vi "TEST - Main Editor VI Not Broken.vi"() -> (0 "error out":errorcluster, 2 "VI not broken? out (true: Pass)":bool)   [LabVIEW 2015]
doc: "Get state of VI to know if is not broken"
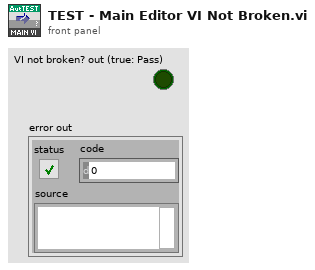
[diagram p1: front panel]
types:
  T1 = enum32{"Bad", "Idle", "Run top level", "Running"}
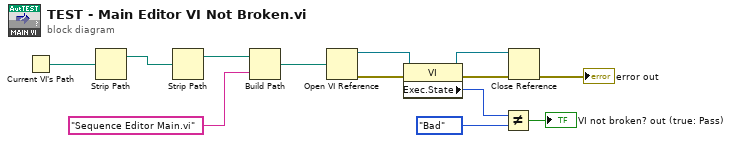
[diagram p0: block diagram]
diagram:
  n1 = Current VI's Path() -> (path=w6:path)
  n2 = Strip Path(path=w6) -> (stripped path=w7:path)  [unwired: 1 out]
  n3 = Strip Path(path=w7) -> (stripped path=w5:path)  [unwired: 1 out]
  n4 = Build Path(base path=w5, name or relative path="Sequence Editor Main.vi") -> (appended path=w3:path)
  n5 = Open VI Reference(vi path=w3) -> (vi reference=w13:refnum<vi>, error out=w12:errorcluster)  [unwired: 5 in]
  n6 = property class="VI"(reference=w13, error in=w12) -> (reference out=w10:refnum<vi>, error out=w11:errorcluster, "Exec.State"=w8:T1)
  n7 = Not Equal?(x=w8, y=T1."Bad" ("Execution:State")) -> (x != y?=→"VI not broken? out (true: Pass)":bool)
  n8 = Close Reference(reference=w10, error in (no error)=w11) -> (error out=→"error out":errorcluster)
